vi "读.vi"(8 "error in (no error)":errorcluster caption="错误输入（无错误）", 11 "通讯 输入":refnum<class "通讯.lvclass">) -> (0 "error out":errorcluster caption="错误输出", 2 "读取缓冲区":string, 3 "通讯 输出":refnum<class "通讯.lvclass">)   [LabVIEW 2015, in "通讯.lvlib" / "通讯.lvclass"]
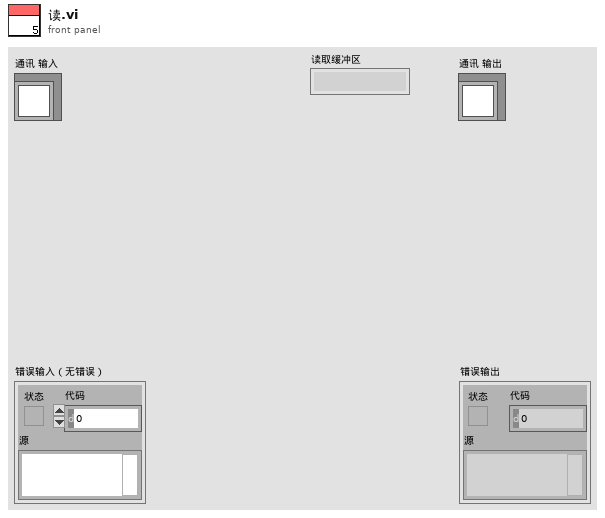
[diagram p1: front panel]
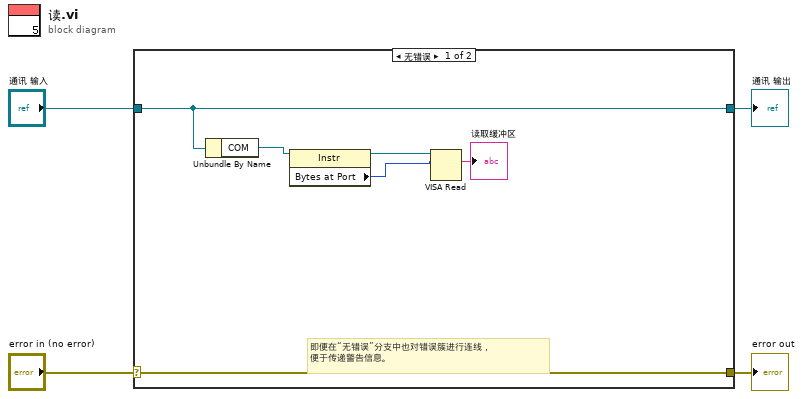
[diagram p0: block diagram]
diagram:
  n1 = case shown="无错误" "error in (no error)" {
    selector: "error in (no error)" -> [w10 w12]
    tunnel: [w10 w12] -> w3
    tunnel: [w9 w11] -> w1
    tunnel: "通讯 输入" -> [w9 w11]
    frame No Error {
      # "即便在“无错误”分支中也对错误簇进行连线，\n便于传递警告信息。"
      n2 = Unbundle By Name(w9) -> ("COM"=w8:refnum<visa-resource-name>)
      n3 = property class="Instr"(reference=w8) -> (reference out=w7:refnum<visa-resource-name>, "Bytes at Port"=w6:u32)  [unwired: 1 in, 1 out]
      n4 = VISA Read(VISA resource name=w7, byte count=w6) -> (read buffer=→"读取缓冲区":string)  [unwired: 1 in, 3 out]
    }
    frame Error {
    }
  }
  "error out" <- w3
  "通讯 输出" <- w1
